vi "state_machine.vi"() -> ()   [LabVIEW 2013]
panel:
  out "stato corrente":string
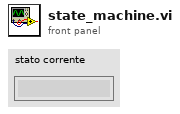
[diagram p1: front panel]
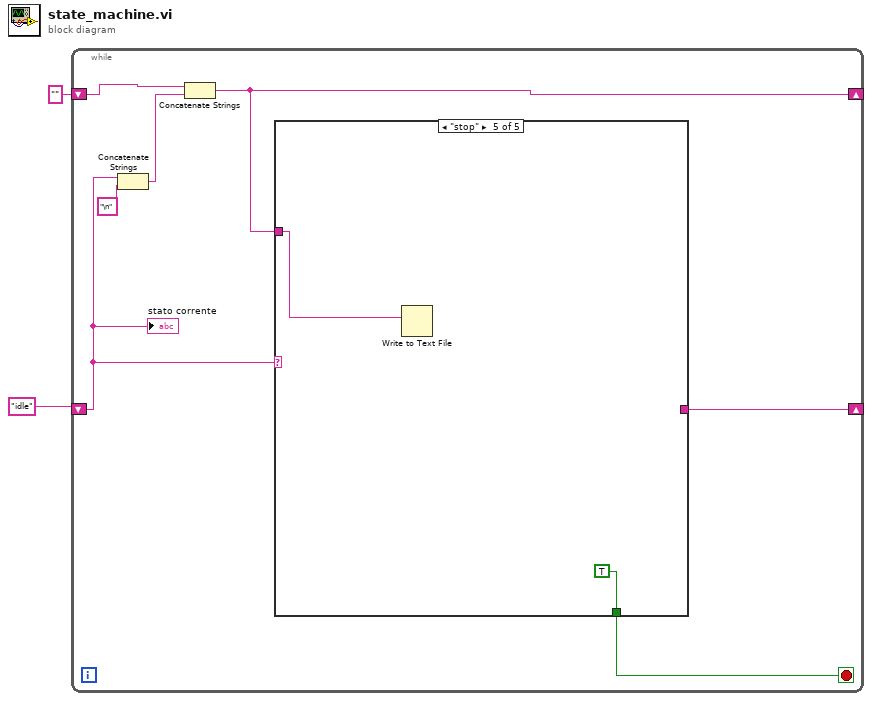
[diagram p0: block diagram]
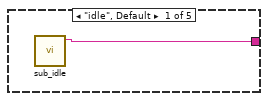
[diagram p2: hidden frame]
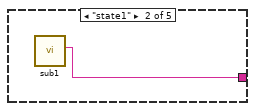
[diagram p3: hidden frame]
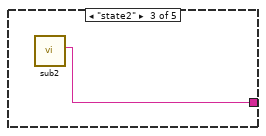
[diagram p4: hidden frame]
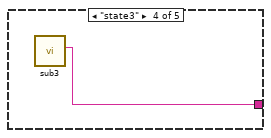
[diagram p5: hidden frame]
diagram:
  n1 = while {
    shift-right: [w8] -> _
    shift-left: "idle" -> [w6]
    shift-right: [w3] -> _
    shift-left: "" -> [w7]
    stop <- w9 stop-if-true
    n2 = Concatenate Strings(w6, "\n" ("string")) -> (w5:string)
    n3 = Concatenate Strings(w7, w5) -> (w3:string)
    n4 = case shown="\"stop\"" w6 {
      tunnel: [_ _ _ _ TRUE] -> w9
      tunnel: [w10 w11 w12 w13 _] -> w8
      tunnel: w3 -> [_ _ _ _ w14]
      frame "idle", Default {
        n5 = call "sub_idle.vi"() -> ("String"=w10:string)  [unwired: 11 in]
      }
      frame "state1" {
        n6 = call "sub1.vi"() -> ("String"=w11:string)  [unwired: 11 in]
      }
      frame "state2" {
        n7 = call "sub2.vi"() -> ("String"=w12:string)  [unwired: 11 in]
      }
      frame "state3" {
        n8 = call "sub3.vi"() -> ("String"=w13:string)  [unwired: 11 in]
      }
      frame "stop" {
        n9 = Write to Text File(text=w14) -> ()  [unwired: 3 in, 3 out]
      }
    }
    "stato corrente" <- w6
  }
